vi "Init.vi"() -> (0 "error out":errorcluster, 3 "ReadOnly":T1={"Qref"={"ValveCTR"=refnum, "Error"=refnum}, "UI_EN"=FALSE, "UserEventREF"={"TimeBasedProducer"={"Reg"=refnum, "Ref"=refnum}, "TimeBasedTempRead"={"Reg"=refnum, "Ref"=refnum}}, "UI_REF"=variant(cluster{} {}), "Paths"={"Log_Dir"=path "", "TempLog"=path "", "WateringLog"=path "", "Error"=path "", "Settings_Dir"=path "", "CFG.ini"=path "", "Plant_Digital_OP"=path "", "TimeTable"=path "", "Consol_Dir"=path "", "Input"=path "", "Output"=path "", "Timeout"=path "", "TimeoutTable"=path "", "Ch_Stat"=path "", "Temp"=path ""}, "PI_REF"={"IO"=enum."Remote", "Interface"=enum."Serial", "LINX Device Config"={"Interface"=enum."Serial", "COM Port"="COM13", "TCP Configuration"={"IP Address"="", "Port"=0}, "Device Family"=1, "Device ID"=1, "Device Name"="myRIO-1900", "TCP Ref"=refnum, "Channels"={"DI"=[0, 1, 2, 3, 4, 5, 6, 7, 8, 9, 10, 11, 12, 13, 14, 15, 16, 17, 18, 19, 20, 21, 22, 23, 24, 25, 26, 27, 28, 29, 30, 31, 32, 33, 34, 35, 36, 37, 38, 39, 40, 41, 42, 43, 44, 45, 46], "DO"=[0, 1, 2, 3, 4, 5, 6, 7, 8, 9, 10, 11, 12, 13, 14, 15, 16, 17, 18, 19, 20, 21, 22, 23, 24, 25, 26, 27, 28, 29, 30, 31, 32, 33, 34, 35, 36, 37, 38, 39, 40, 41, 42, 43, 44, 45, 46], "AI"=[0, 1, 2, 3, 4, 5, 6, 7, 8, 9, 10, 11], "AO"=[], "PWM"=[3, 5, 6, 9, 10], "QE"=[], "UART"=[0, 1], "I2C 2"=[0], "SPI"=[0], "CAN"=[], "Servo"=[], "AI Ref (V)"=0.0, "AI Resolution (Bits)"=0, "AO Ref (V)"=0.0, "AO Resolution (Bits)"=0}}}, "CFG"={"ProducerEn_PC"=FALSE, "Producer_PC_ms"=0, "ProducerEn_PI"=FALSE, "Producer_PI_ms"=0, "TempLogInterval"=15, "SystemResetTime"=0.0}} {"CFG"."SystemResetTime" format="%<%H:%M:%S>t"})   [LabVIEW 2014, in "Main.lvlib"]
uses:
  Main.lvlib
  TypeDef/ReadOnly.ctl
  ValveCTRL/TypeDef/Queue_Cluster.ctl
  ValveCTRL/TypeDef/States_Enum.ctl
  ValveCTRL/TypeDef/CHs_List.ctl
  TypeDef/EventData.ctl
  <vilib>/MakerHub/LINX/Private/Type Defs/LINX Ref.ctl
  <vilib>/MakerHub/LINX/Private/Type Defs/Platform.ctl
  <vilib>/MakerHub/LINX/Private/Type Defs/Interface.ctl
  <vilib>/MakerHub/LINX/Private/Device/Type Defs/LINX Device Config.ctl
  <vilib>/MakerHub/LINX/Private/Device/Type Defs/TCP Config.ctl
  <vilib>/MakerHub/LINX/Private/Device/Type Defs/Channels.ctl
  ReadInitCFG/TypeDef/CFG_Cluster.ctl
  <vilib>/MakerHub/LINX/Public/Utilities/Open Local.vi
  <vilib>/MakerHub/LINX/LMH-LINX.lvlib
  ValveCTRL/ValveCTRL.lvlib
  <vilib>/MakerHub/LINX/Private/Device/Device.lvlib
  Files_OP/Files_OP.lvlib
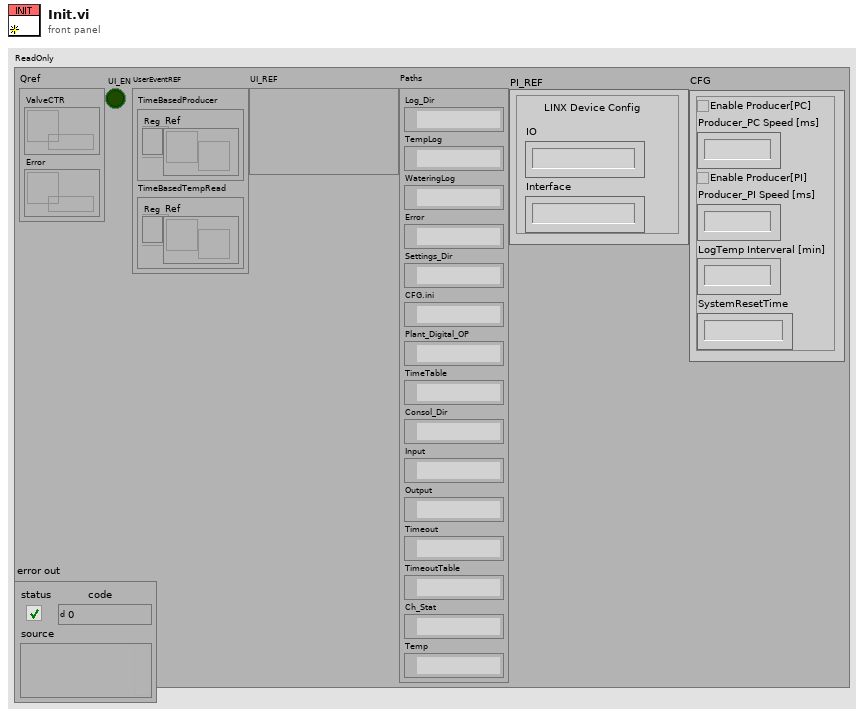
[diagram p1: front panel]
types:
  T1 = typedef "Main.lvlib/ReadOnly.ctl" = cluster{"Qref":cluster{"ValveCTR":refnum<queue>, "Error":refnum<queue>}, "UI_EN":bool, "UserEventREF":cluster{"TimeBasedProducer":cluster{"Reg":refnum<event-registration>, "Ref":refnum<user-event>}, "TimeBasedTempRead":cluster{"Reg":refnum<event-registration>, "Ref":refnum<user-event>}}, "UI_REF":variant, "Paths":cluster{"Log_Dir":path, "TempLog":path, "WateringLog":path, "Error":path, "Settings_Dir":path, "CFG.ini":path, "Plant_Digital_OP":path, "TimeTable":path, "Consol_Dir":path, "Input":path, "Output":path, "Timeout":path, "TimeoutTable":path, "Ch_Stat":path, "Temp":path}, "PI_REF":T2, "CFG":T8}
  T2 = typedef "LMH-LINX.lvlib/LINX Ref.ctl" = cluster{"IO":T3, "Interface":T4, "LINX Device Config":T5}
  T3 = typedef "LMH-LINX.lvlib/Platform.ctl" = enum16{"Remote", "Local"}
  T4 = typedef "LMH-LINX.lvlib/Interface.ctl" = enum16{"Serial", "TCP"}
  T5 = typedef "LMH-LINX.lvlib/Device.lvlib/LINX Device Config.ctl" = cluster{"Interface":T4, "COM Port":refnum<visa-resource-name>, "TCP Configuration":T6, "Device Family":u8, "Device ID":u8, "Device Name":string, "TCP Ref":refnum<k5>, "Channels":T7}
  T6 = typedef "LMH-LINX.lvlib/Device.lvlib/TCP Config.ctl" = cluster{"IP Address":string, "Port":u16}
  T7 = typedef "LMH-LINX.lvlib/Channels.ctl" = cluster{"DI":u8[], "DO":u8[], "AI":u8[], "AO":u8[], "PWM":u8[], "QE":u8[], "UART":u8[], "I2C 2":u8[], "SPI":u8[], "CAN":u8[], "Servo":u8[], "AI Ref (V)":dbl, "AI Resolution (Bits)":u8, "AO Ref (V)":dbl, "AO Resolution (Bits)":u8}
  T8 = typedef "Main.lvlib/CFG_Cluster.ctl" = cluster{"ProducerEn_PC":bool, "Producer_PC_ms":u32, "ProducerEn_PI":bool, "Producer_PI_ms":u32, "TempLogInterval":u32, "SystemResetTime":dbl}
  T9 = typedef "Main.lvlib/EventData.ctl" = cluster{"State":string, "Data":variant}
  T10 = typedef "ValveCTRL.lvlib/Queue_Cluster.ctl" = cluster{"State":T11, "Channel No":T12, "Duration[S]":dbl}
  T11 = typedef "ValveCTRL.lvlib/States_Enum.ctl" = enum16{"Open Pump", "Open Valve", "Wait Valve", "Close Pump", "Close Valve", "Save State", "StopLoop", "ValidCh"}
  T12 = typedef "ValveCTRL.lvlib/CHs_List.ctl" = u8
  T13 = enum16{"open", "replace", "create", "open or create", "replace or create", "replace or create with confirmation"}
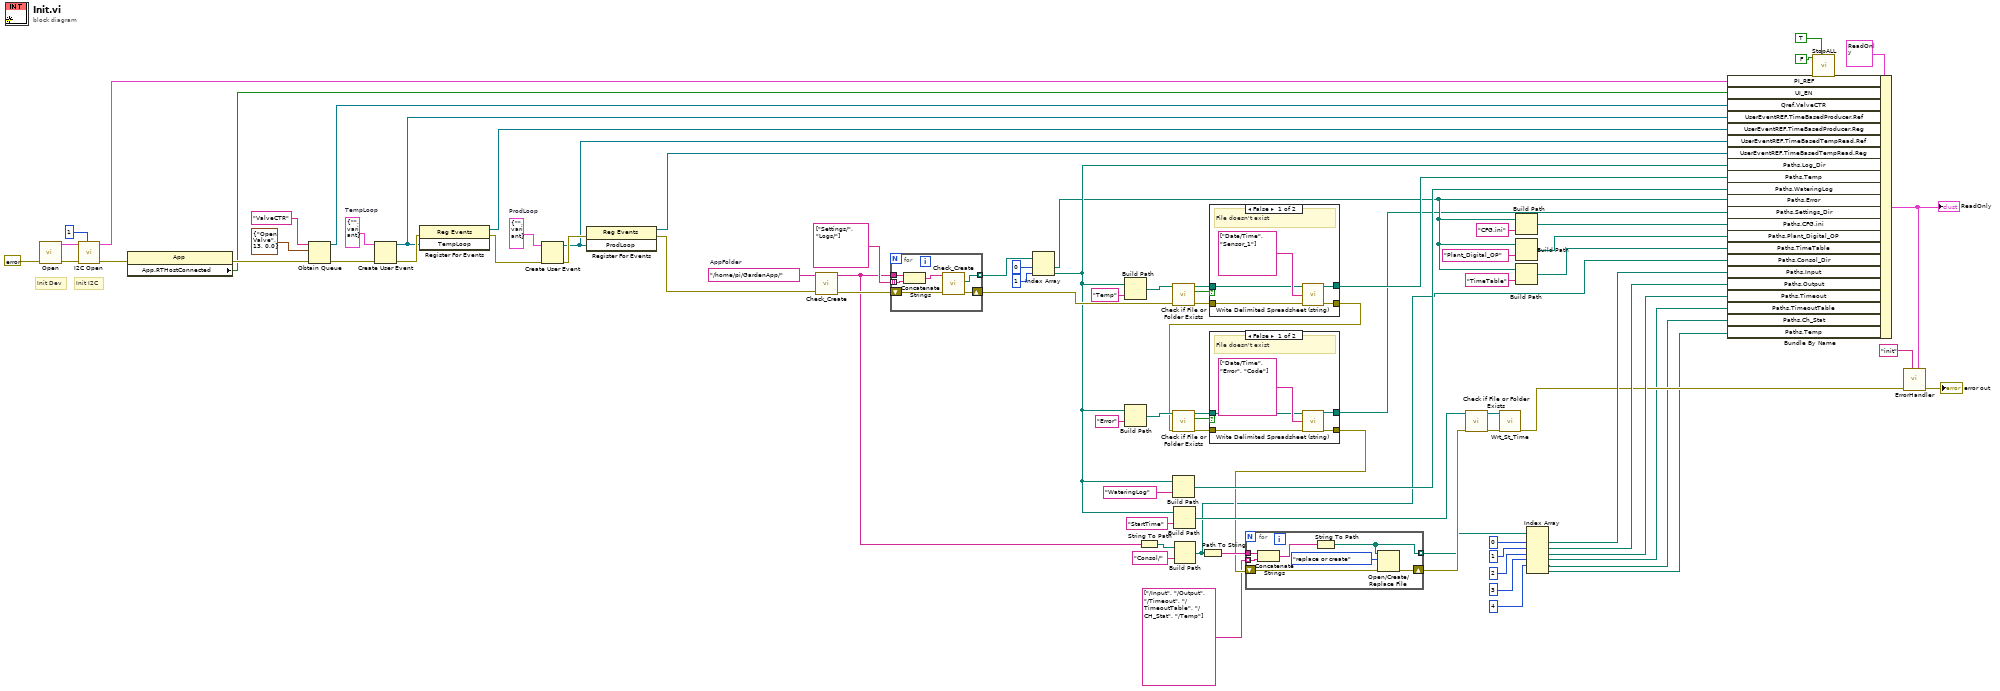
[diagram p0: block diagram]
diagram:
  w63 = "/home/pi/GardenApp/"  # AppFolder
  w73 = T9 {"State"="", "Data"=variant}  # ProdLoop
  w74 = T9 {"State"="", "Data"=variant}  # TempLoop
  # "Init I2C"
  # "Init Dev"
  n1 = call-poly <vilib>:"Open.vi"("Error In"=errorcluster {"status"=FALSE, "code"=0, "source"=""}) -> ("Error Out"=w82:errorcluster, "LINX Resource"=w81:T2)  [unwired: 8 in, 1 out]
  n2 = call <vilib>:"I2C Open.vi"("I2C Channel (0)"=u8 1, "Error In"=w82, "LINX Resource"=w81) -> ("Error Out"=w12:errorcluster, "LINX Resource"=w75:T2)  [unwired: 7 in]
  n3 = property class="App"(error in=w12) -> (error out=w11:errorcluster, "App.RTHostConnected"=w10:bool)  [unwired: 1 in, 1 out]
  n4 = Obtain Queue(name (unnamed)="ValveCTR", element data type=T10 {"State"=enum."Open Valve", "Channel No"=13, "Duration[S]"=0.0} ("ValveCTRL"), error in (no error)=w11) -> (queue out=w76:refnum<queue>, error out=w70:errorcluster)  [unwired: 2 in, 1 out]
  n5 = Create User Event(user event datatype=w74, error in=w70) -> (user event=w69:refnum<user-event>, error out=w72:errorcluster)
  n6 = register-events(error in=w72, w69) -> (reference out=w68:refnum<event-registration>, error out=w67:errorcluster)  [unwired: 1 in]
  n7 = Create User Event(user event datatype=w73, error in=w67) -> (user event=w66:refnum<user-event>, error out=w71:errorcluster)
  n8 = register-events(error in=w71, w66) -> (reference out=w65:refnum<event-registration>, error out=w64:errorcluster)  [unwired: 1 in]
  n9 = call "Check_Create.vi"("error in"=w64, "PathIn"=w63) -> ("error out"=w62:errorcluster, "PathOut"=w27:string)  [unwired: 7 in, 1 out]
  n10 = for {
    shift-right: [w88] -> w51
    shift-left: w62 -> [w89]
    tunnel: w27 -> [w86]
    tunnel: string[] ["Settings/", "Logs/"] -> [w85] mode=indexing
    tunnel: [w84] -> w60 mode=indexing
    n11 = Concatenate Strings(w86, w85) -> (w87:string)
    n12 = call "Check_Create.vi"("error in"=w89, "PathIn"=w87) -> ("error out"=w88:errorcluster, "dup path"=w84:path)  [unwired: 7 in, 1 out]
  }
  n13 = Index Array(array=w60, index #1=0 ("index"), index #2=1 ("index")) -> (element #1=w33:path, element #2=w35:path)
  n14 = Build Path(base path=w35, name or relative path="Temp") -> (appended path=w56:path)
  n15 = Build Path(base path=w35, name or relative path="Error") -> (appended path=w37:path)
  n16 = String To Path(string=w27) -> (path=w28:path)
  n17 = call <vilib>:"Check if File or Folder Exists.vi"("error in (no error)"=w51, "path"=w56) -> ("error out"=w54:errorcluster, "file or folder exists?"=w55:bool, "dup path"=w53:path)  [unwired: 7 in]
  n18 = Build Path(base path=w35, name or relative path="WateringLog") -> (appended path=w46:path)
  n19 = Build Path(base path=w35, name or relative path="StartTime") -> (appended path=w52:path)
  n20 = Build Path(base path=w28, name or relative path="Consol/") -> (appended path=w22:path)
  n21 = Path To String(path=w22) -> (string=w26:string)
  n22 = case shown="False" w55 {
    tunnel: w54 -> [w94 w96]
    tunnel: w53 -> [w92 w95]
    tunnel: [w91 w96] -> w34
    tunnel: [w90 w95] -> w45
    frame False {
      # "File doesn't exist"
      n23 = call "Write Delimited Spreadsheet (string).vi"("file path (dialog if empty)"=w92, "1D data"=string[] ["Date/Time", "Sensor_1"], "error in (no error)"=w94) -> ("new file path (Not A Path if cancelled)"=w90:path, "error out"=w91:errorcluster)  [unwired: 11 in]
    }
    frame True {
    }
  }
  n24 = call <vilib>:"Check if File or Folder Exists.vi"("error in (no error)"=w34, "path"=w37) -> ("error out"=w39:errorcluster, "file or folder exists?"=w38:bool, "dup path"=w40:path)  [unwired: 7 in]
  n25 = case shown="False" w38 {
    tunnel: w39 -> [w101 w103]
    tunnel: w40 -> [w99 w102]
    tunnel: [w98 w103] -> w25
    tunnel: [w97 w102] -> w31
    frame False {
      # "File doesn't exist"
      n26 = call "Write Delimited Spreadsheet (string).vi"("file path (dialog if empty)"=w99, "1D data"=string[] ["Date/Time", "Error", "Code"], "error in (no error)"=w101) -> ("new file path (Not A Path if cancelled)"=w97:path, "error out"=w98:errorcluster)  [unwired: 11 in]
    }
    frame True {
    }
  }
  n27 = for {
    shift-right: [w107] -> w23
    shift-left: w25 -> [w106]
    tunnel: w26 -> [w110]
    tunnel: string[] ["/Input", "/Output", "/Timeout", "/TimeoutTable", "/CH_Stat", "/Temp"] -> [w109] mode=indexing
    tunnel: [w104] -> w17 mode=indexing
    n28 = Concatenate Strings(w110, w109) -> (w105:string)
    n29 = String To Path(string=w105) -> (path=w104:path)
    n30 = Open/Create/Replace File(file path (use dialog)=w104, error in=w106, operation (0:open)=T13."replace or create") -> (error out=w107:errorcluster)  [unwired: 3 in, 2 out]
  }
  n31 = call <vilib>:"Check if File or Folder Exists.vi"("error in (no error)"=w23, "path"=w52) -> ("error out"=w49:errorcluster, "dup path"=w48:path)  [unwired: 7 in, 1 out]
  n32 = call "Wrt_St_Time.vi"("Error In"=w49, "StartTimePath"=w48) -> ("Error Out"=w8:errorcluster)  [unwired: 9 in]
  n33 = Build Path(base path=w33, name or relative path="CFG.ini") -> (appended path=w43:path)
  n34 = Build Path(base path=w33, name or relative path="Plant_Digital_OP") -> (appended path=w32:path)
  n35 = Build Path(base path=w33, name or relative path="TimeTable") -> (appended path=w30:path)
  n36 = Index Array(array=w17, index #1=0 ("index"), index #2=1 ("index"), index #3=2 ("index"), index #4=3 ("index"), index #5=4 ("index")) -> (element #1=w19:path, element #2=w18:path, element #3=w13:path, element #4=w4:path, element #5=w3:path, element #6=w1:path)  [unwired: 1 in]
  n37 = Bundle By Name(cluster=T1 {"Qref"={"ValveCTR"=refnum, "Error"=refnum}, "UI_EN"=FALSE, "UserEventREF"={"TimeBasedProducer"={"Reg"=refnum, "Ref"=refnum}, "TimeBasedTempRead"={"Reg"=refnum, "Ref"=refnum}}, "UI_REF"=variant(cluster{} {}), "Paths"={"Log_Dir"=path "", "TempLog"=path "", "WateringLog"=path "", "Error"=path "", "Settings_Dir"=path "", "CFG.ini"=path "", "Plant_Digital_OP"=path "", "TimeTable"=path "", "Consol_Dir"=path "", "Input"=path "", "Output"=path "", "Timeout"=path "", "TimeoutTable"=path "", "Ch_Stat"=path "", "Temp"=path ""}, "PI_REF"={"IO"=enum."Remote", "Interface"=enum."Serial", "LINX Device Config"={"Interface"=enum."Serial", "COM Port"="COM13", "TCP Configuration"={"IP Address"="", "Port"=0}, "Device Family"=1, "Device ID"=1, "Device Name"="myRIO-1900", "TCP Ref"=refnum, "Channels"={"DI"=[0, 1, 2, 3, 4, 5, 6, 7, 8, 9, 10, 11, 12, 13, 14, 15, 16, 17, 18, 19, 20, 21, 22, 23, 24, 25, 26, 27, 28, 29, 30, 31, 32, 33, 34, 35, 36, 37, 38, 39, 40, 41, 42, 43, 44, 45, 46], "DO"=[0, 1, 2, 3, 4, 5, 6, 7, 8, 9, 10, 11, 12, 13, 14, 15, 16, 17, 18, 19, 20, 21, 22, 23, 24, 25, 26, 27, 28, 29, 30, 31, 32, 33, 34, 35, 36, 37, 38, 39, 40, 41, 42, 43, 44, 45, 46], "AI"=[0, 1, 2, 3, 4, 5, 6, 7, 8, 9, 10, 11], "AO"=[], "PWM"=[3, 5, 6, 9, 10], "QE"=[], "UART"=[0, 1], "I2C 2"=[0], "SPI"=[0], "CAN"=[], "Servo"=[], "AI Ref (V)"=0.0, "AI Resolution (Bits)"=0, "AO Ref (V)"=0.0, "AO Resolution (Bits)"=0}}}, "CFG"={"ProducerEn_PC"=FALSE, "Producer_PC_ms"=0, "ProducerEn_PI"=FALSE, "Producer_PI_ms"=0, "TempLogInterval"=15, "SystemResetTime"=0.0}} ("ReadOnly"), "PI_REF"=w75, "UI_EN"=w10, "Qref.ValveCTR"=w76, "UserEventREF.TimeBasedProducer.Ref"=w69, "UserEventREF.TimeBasedProducer.Reg"=w68, "UserEventREF.TimeBasedTempRead.Ref"=w66, "UserEventREF.TimeBasedTempRead.Reg"=w65, "Paths.Log_Dir"=w35, "Paths.Temp"=w45, "Paths.WateringLog"=w46, "Paths.Error"=w31, "Paths.Settings_Dir"=w33, "Paths.CFG.ini"=w43, "Paths.Plant_Digital_OP"=w32, "Paths.TimeTable"=w30, "Paths.Consol_Dir"=w22, "Paths.Input"=w19, "Paths.Output"=w18, "Paths.Timeout"=w13, "Paths.TimeoutTable"=w4, "Paths.Ch_Stat"=w3, "Paths.Temp"=w1) -> (w9:T1)
  "ReadOnly" <- w9
  n38 = call "StopALL.vi"("Write[F]"=TRUE, "StopIN"=FALSE) -> ()  [unwired: 9 in, 1 out]
  n39 = call "ErrorHandler.vi"("ReadOnlyIn"=w9, "LoopName"="init", "error in"=w8) -> ("error out"=→"error out":errorcluster)  [unwired: 8 in]
